vi "Init UI.vi"(8 "error in (no error)":errorcluster, 11 "UI VISA Terminal in":refnum<class "UI VISA Terminal.lvclass">) -> (0 "error out":errorcluster, 3 "UI VISA Terminal out":refnum<class "UI VISA Terminal.lvclass">)   [LabVIEW 2025, in "UI VISA Terminal.lvlib" / "UI VISA Terminal.lvclass"]
uses:
  UI VISA Terminal.lvclass
  UI VISA Terminal.lvclass/UI VISA Terminal.ctl
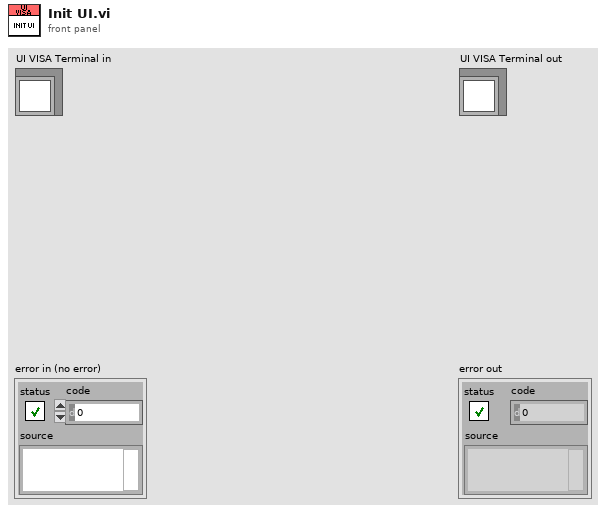
[diagram p1: front panel]
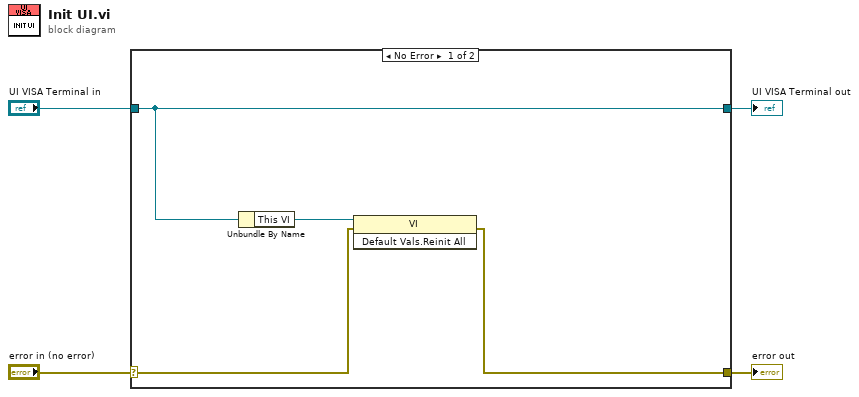
[diagram p0: block diagram]
diagram:
  n1 = case shown="No Error" "error in (no error)" {
    selector: "error in (no error)" -> [w6 w10]
    tunnel: [w5 w10] -> w3
    tunnel: [w8 w9] -> w1
    tunnel: "UI VISA Terminal in" -> [w8 w9]
    frame No Error {
      n2 = Unbundle By Name(w8) -> ("This VI"=w7:refnum<vi>)
      n3 = invoke class="VI" method="Default Vals.Reinit All"(reference=w7, error in=w6) -> (error out=w5:errorcluster)  [unwired: 1 in, 2 out]
    }
    frame Error {
    }
  }
  "error out" <- w3
  "UI VISA Terminal out" <- w1
